vi "Periodic Tasks.vi"(8 "error in":errorcluster) -> ()   [LabVIEW 2017]
doc: "This VI runs in parallel to other tasks. It can contain as many user-defined periodic loops as you need. These can carry out PID or other sorts of timed response."
uses:
  <vilib>/Rock Robotics/WPI/SerialPort/WPI_SerialPort.ctl
  <vilib>/Rock Robotics/WPI/Utilities/WPI_GetSetVariantRefNum.vi
  <vilib>/Rock Robotics/WPI/Ultrasonic/WPI_SonarMB1010AnalogRefNum Registry Get.vi
  Robot Global Data.vi
  <vilib>/Rock Robotics/WPI/Ultrasonic/WPI_SonarMB1010AnalogGetRange.vi
  <vilib>/Rock Robotics/Network Tables/NT Write Number.vi
  <vilib>/Rock Robotics/Network Tables/NT Write Numeric Array.vi
panel:
  out "Blinky":bool
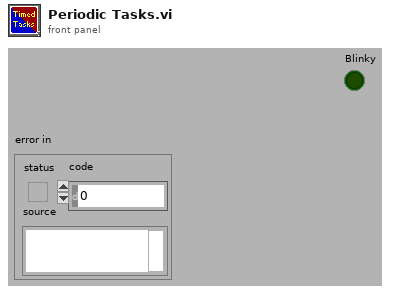
[diagram p1: front panel]
types:
  T1 = typedef "WPI_SonarMB1010AnalogDeviceRef.ctl" = cluster{"AIDeviceRef":T2, "Scaling factor (V/in)":dbl, "Average Bits":u8}
  T2 = typedef "WPI_AnalogChannelDevRef.ctl" = cluster{"DevStatus":errorcluster, "Analog Channel":T3}
  T3 = typedef "FPGA_AIChannel.ctl" = enum8{"AI 0", "AI 1", "AI 2", "AI 3", "AI MXP 0", "AI MXP 1", "AI MXP 2", "AI MXP 3", "Invalid"}
  T4 = typedef "WPI_DigitalInputDevRef.ctl" = cluster{"DevStatus":errorcluster, "DIO Channel":T5}
  T5 = typedef "FPGA_DIOChannel.ctl" = enum8{"DIO 0", "DIO 1", "DIO 2", "DIO 3", "DIO 4", "DIO 5", "DIO 6", "DIO 7", "DIO 8", "DIO 9", "DIO MXP 0", "DIO MXP 1", "DIO MXP 2", "DIO MXP 3", "DIO MXP 4", "DIO MXP 5", "DIO MXP 6", "DIO MXP 7", "DIO MXP 8", "DIO MXP 9", "DIO MXP 10", "DIO MXP 11", "DIO MXP 12", "DIO MXP 13", "DIO MXP 14", "DIO MXP 15", "SPI Port CS1", "SPI Port CS2", "SPI Port CS3", "SPI Port MISO", "SPI Port MOSI", "Invalid"}
  T6 = typedef "WPI_GyroDevRef.ctl" = cluster{"DevStatus":errorcluster, "Analog Channel":T3, "Gain (VoltsPerDegree/Second)":dbl, "Gyro Type":enum16{"Analog", "XRS450"}, "Handle":i32, "SPI Bus":T7, "Device Found":bool, "Sample Rate":dbl, "Calibrate On Open":bool, "Offset":dbl}
  T7 = typedef "spi_bus.ctl" = enum16{"SPI On-Board, CS0", "SPI On-Board, CS1", "SPI On-Board, CS2", "SPI On-Board, CS3", "SPI MXP", "Invalid"}
  T8 = typedef "WPI_JoystickDevRef.ctl" = cluster{"Device":T9}
  T9 = typedef "WPI_JoystickDeviceEnum.ctl" = enum16{"USB 0", "USB 1", "USB 2", "USB 3", "USB 4", "USB 5"}
  T10 = cluster{"GyroDevRef":T6, "JoystickDevRef":T8, "SonarMB1010AnalogDevRef":T1, "DigitalInputDevRef":T4}
  T11 = cluster{"Yaw":dbl, "Roll":dbl, "Pitch":dbl, "Heading":dbl, "Fused Heading":dbl}
  T12 = typedef "WPI_SerialPort.ctl" = enum16{"Onboard RS-232", "MXP TTL", "USB 1", "USB 2"}
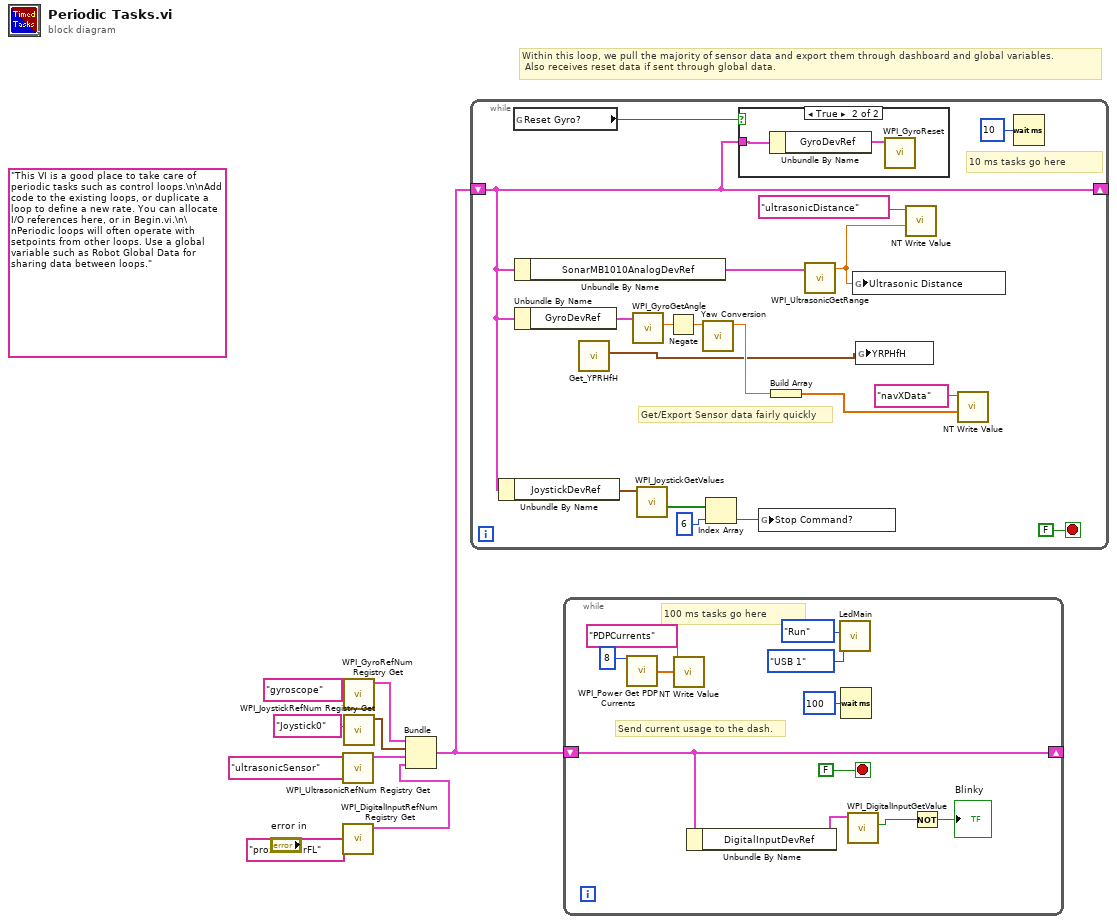
[diagram p0: block diagram]
diagram:
  (unwired) "This VI is a good place to take care of periodic tasks such as control loops.\n\nAdd code to the existing loops, or duplicate a loop to define a new rate. You can allocate I/O references here, or in Begin.vi.\n\nPeriodic loops will often operate with setpoints from other loops. Use a global variable such as Robot Global Data for sharing data between loops."
  # "Within this loop, we pull the majority of sensor data and export them through dashboard and global variables.\n Also receives reset data if sent through global data."
  n1 = call-poly <vilib>:"WPI_UltrasonicRefNum Registry Get.vi"("refnum name"="ultrasonicSensor") -> ("SonarMB1010AnalogDevRef"=w4:T1)  [unwired: 9 in, 1 out]
  n2 = call <vilib>:"WPI_DigitalInputRefNum Registry Get.vi"("refnum name"="proxSensorFL") -> ("DigitalInputDevRef"=w2:T4)  [unwired: 9 in, 1 out]
  n3 = call <vilib>:"WPI_GyroRefNum Registry Get.vi"("refnum name"="gyroscope") -> ("GyroDevRef"=w5:T6)  [unwired: 9 in, 1 out]
  n4 = call <vilib>:"WPI_JoystickRefNum Registry Get.vi"("refnum name"="Joystick0") -> ("JoystickDevRef"=w9:T8)  [unwired: 9 in, 1 out]
  n5 = Bundle("GyroDevRef"=w5, "JoystickDevRef"=w9, "SonarMB1010AnalogDevRef"=w4, "DigitalInputDevRef"=w2) -> (w7:T10)  [unwired: 1 out]
  n6 = while {
    shift-right: [w21] -> _
    shift-left: w7 -> [w21]
    stop <- FALSE stop-if-true
    # "Get/Export Sensor data fairly quickly"
    # "10 ms tasks go here"
    n7 = Unbundle By Name(w21) -> ("JoystickDevRef"=w20:T8)
    n8 = global read "Robot Global Data.vi" "Reset Gyro?"() -> (w22:bool)
    n9 = Unbundle By Name(w21) -> ("SonarMB1010AnalogDevRef"=w13:T1)
    n10 = Unbundle By Name(w21) -> ("GyroDevRef"=w24:T6)
    n11 = call <vilib>:"Get_YPRHfH.vi"() -> ("YRPHfH"=w10:T11)  [unwired: 11 in]
    n12 = call <vilib>:"WPI_GyroGetAngle.vi"("GyroDevRef"=w24) -> ("Angle"=w14:dbl)  [unwired: 6 in, 4 out]
    n13 = call <vilib>:"WPI_JoystickGetValues.vi"("JoystickDevRef"=w20) -> ("Buttons"=w19:bool[])  [unwired: 6 in, 4 out]
    n14 = Negate(x=w14) -> (-x=w16:dbl)
    n15 = call "Yaw Conversion.vi"("Input"=w16) -> ("Output"=w15:dbl)  [unwired: 10 in]
    n16 = Index Array(array=w19, index=6) -> (element=w17:bool)
    n17 = case shown="True" w22 {
      tunnel: w21 -> [_ w29]
      frame False {
      }
      frame True {
        n18 = Unbundle By Name(w29) -> ("GyroDevRef"=w28:T6)
        n19 = call <vilib>:"WPI_GyroReset.vi"("GyroDevRef"=w28) -> ()  [unwired: 9 in, 2 out]
      }
    }
    n20 = global write "Robot Global Data.vi" "Stop Command?"(w17) -> ()
    n21 = Build Array(w15) -> (w23:dbl[])
    n22 = call-poly <vilib>:"WPI_UltrasonicGetRange.vi"("SonarMB1010AnalogDevRef"=w13) -> ("Distance"=w12:dbl)  [unwired: 8 in, 2 out]
    n23 = global write "Robot Global Data.vi" "Ultrasonic Distance"(w12) -> ()
    n24 = global write "Robot Global Data.vi" "YRPHfH"(w10) -> ()
    n25 = call-poly <vilib>:"NT Write Value.vi"("Numeric"=w12, "Name"="ultrasonicDistance") -> ()  [unwired: 9 in, 1 out]
    n26 = call-poly <vilib>:"NT Write Value.vi"("Numeric Array"=w23, "Name"="navXData") -> ()  [unwired: 9 in, 1 out]
    n27 = Wait (ms)(milliseconds to wait=u32 10) -> ()  [unwired: 1 out]
  }
  n28 = while {
    shift-right: [w32] -> _
    shift-left: w7 -> [w32]
    stop <- FALSE stop-if-true
    # "Send current usage to the dash."
    # "100 ms tasks go here"
    n29 = call <vilib>:"WPI_Power Get PDP Currents.vi"("Power Distribution Panel (0)"=u8 8) -> ("all currents (A)"=w38:dbl[])  [unwired: 12 in, 2 out]
    n30 = call-poly <vilib>:"NT Write Value.vi"("Numeric Array"=w38, "Name"="PDPCurrents") -> ()  [unwired: 9 in, 1 out]
    n31 = Unbundle By Name(w32) -> ("DigitalInputDevRef"=w33:T4)
    n32 = call "LedMain.vi"("Serial Port"=WPI_SerialPort."USB 1", "Mode"=enum16{"Open", "Run"}."Run") -> ()  [unwired: 10 in]
    n33 = Wait (ms)(milliseconds to wait=u32 100) -> ()  [unwired: 1 out]
    n34 = call <vilib>:"WPI_DigitalInputGetValue.vi"("DigitalInputDevRef"=w33) -> ("Value"=w31:bool)  [unwired: 8 in, 2 out]
    n35 = Not(x=w31) -> (.not. x?=→"Blinky":bool)
  }
